vi "Check File Size.vi"(8 "error in":errorcluster, 11 "File Actor in":refnum<class "File Actor.lvclass">) -> (0 "error out":errorcluster, 3 "File Actor out":refnum<class "File Actor.lvclass">)   [LabVIEW 2014, in "File Library.lvlib" / "File Actor.lvclass"]
doc: "Checks the current file size. If his value exceeds the specified maximum, then a message will be sent to indicate that the file needs to be changed."
uses:
  File Actor.lvclass
  File Actor.lvclass/File Actor.ctl
  Messages/To/Change File MSG/Change File MSG.lvclass
  <vilib>/ActorFramework/Actor/Actor.lvclass/Actor.ctl
  <vilib>/ActorFramework/Message Enqueuer/Message Enqueuer.lvclass/Message Enqueuer.ctl
  <vilib>/ActorFramework/Message Enqueuer/Init from Existing Queue.vi
  <vilib>/ActorFramework/Message Priority Queue/Priority Enqueue.vi
  <vilib>/ActorFramework/Message Enqueuer/Message Enqueuer.lvclass
  <vilib>/ActorFramework/Actor/Actor.lvclass
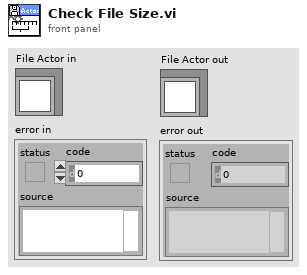
[diagram p1: front panel]
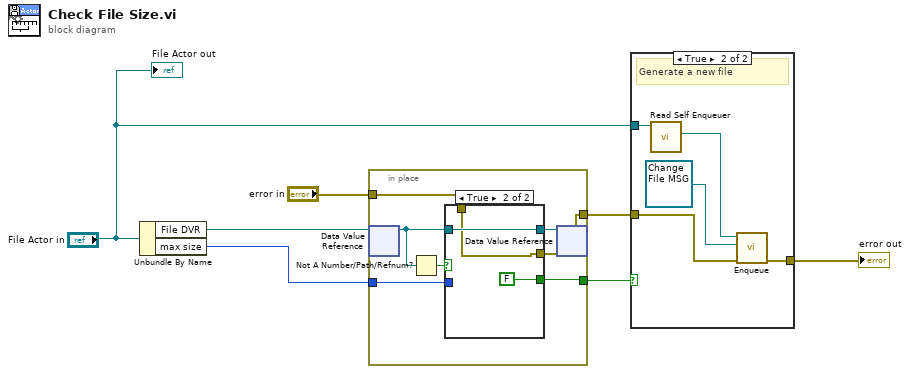
[diagram p0: block diagram]
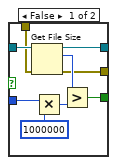
[diagram p3: hidden frame]
diagram:
  n1 = Unbundle By Name("File Actor in") -> ("File DVR"=w7:refnum<data-value>, "max size"=w6:i32)
  n2 = in-place {
    in-place-border: w6 -> [w14]
    in-place-border: [w12] -> w4
    in-place-border: "error in" -> [w9]
    in-place-border: [w8] -> w2
    n3 = in-place-dvr #1(w7) -> (w11:refnum<file>)  [unwired: 1 out]
    n4 = Not A Number/Path/Refnum?(number/path/refnum=w11) -> (NaN/Path/Refnum?=w10:bool)
    n5 = case shown="True" w10 {
      tunnel: w14 -> [w23 _]
      tunnel: [w21 w26] -> w13
      tunnel: [w18 FALSE] -> w12
      tunnel: w11 -> [w17 w26]
      tunnel: w9 -> [w16 w24]
      tunnel: [w15 w24] -> w8
      frame False {
        n6 = Get File Size(file=w17, error in=w16) -> (refnum out=w21:refnum<file>, size (in bytes)=w19:i64, 0:w15:errorcluster)
        n7 = Multiply(x=w23, y=1000000) -> (x*y=w20:i32)
        n8 = Greater?(x=w19, y=w20) -> (0:w18:bool)
      }
      frame True {
      }
    }
    n9 = in-place-dvr #1(w13) -> ()  [unwired: 2 out]
  }
  n10 = case shown="True" w4 {
    tunnel: "File Actor in" -> [_ w32]
    tunnel: w2 -> [w27 w29]
    tunnel: [w27 w28] -> w1
    frame False {
    }
    frame True {
      # "Generate a new file"
      n11 = call <vilib>:"Read Self Enqueuer.vi"("Actor"=w32) -> ("Self Enqueuer"=w31:refnum<class "Message Enqueuer.lvclass">)  [unwired: 10 in]
      n12 = call <vilib>:"Enqueue.vi"("error in (no error)"=w29, "Message"=refnum<class "Change File MSG.lvclass"> refnum ("File Library.lvlib:Change File MSG"), "Message Enqueuer in"=w31) -> ("error out"=w28:errorcluster)  [unwired: 7 in, 1 out]
    }
  }
  "error out" <- w1
  "File Actor out" <- "File Actor in"
